vi "API Value to Temp.vi"(10 "API Temp":dbl) -> (2 "Color Temp":dbl)   [LabVIEW 2022 SP3, in "TouchControl.lvlib" / "LightsPanel.lvclass"]
uses:
  LightsPanel.lvclass
  <vilib>/Analysis/NI_AALPro.lvlib
panel:
  out "offset":dbl
  out "power":dbl
  out "amplitude":dbl
  out "Best Power Fit":dbl[](array[numeric])
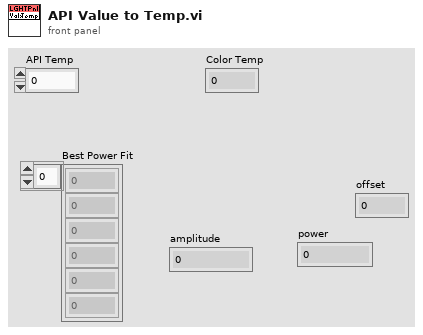
[diagram p1: front panel]
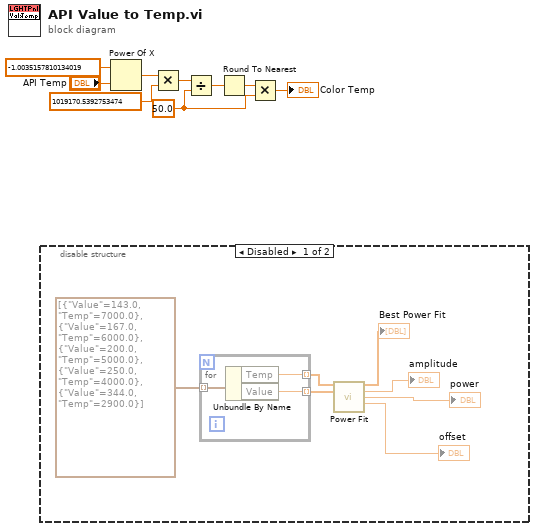
[diagram p0: block diagram]
diagram:
  w1 = 50.0 ("y")
  n1 = disable-structure shown="Disabled" {
    frame Disabled {
      n2 = for {
        tunnel: cluster{"Value":dbl, "Temp":dbl}[] [{"Value"=143.0, "Temp"=7000.0}, {"Value"=167.0, "Temp"=6000.0}, {"Value"=200.0, "Temp"=5000.0}, {"Value"=250.0, "Temp"=4000.0}, {"Value"=344.0, "Temp"=2900.0}] -> [w19] mode=indexing
        tunnel: [w18] -> w15 mode=indexing
        tunnel: [w17] -> w14 mode=indexing
        n3 = Unbundle By Name(w19) -> ("Temp"=w18:dbl, "Value"=w17:dbl)
      }
      n4 = call <vilib>:"Power Fit.vi"("Y"=w15, "X"=w14) -> ("Best Power Fit"=→"Best Power Fit":dbl[], "amplitude"=→"amplitude":dbl, "power"=→"power":dbl, "offset"=→"offset":dbl)  [unwired: 8 in, 2 out]
    }
    frame Enabled {
    }
  }
  n5 = Power Of X(1:"API Temp", 2:-1.0035157810134019 ("power")) -> (0:w5:dbl)
  n6 = Multiply(x=w5, y=1019170.5392753474) -> (x*y=w8:dbl)
  n7 = Divide(x=w8, y=w1) -> (x/y=w4:dbl)
  n8 = Round To Nearest(number=w4) -> (nearest integer value=w3:dbl)
  n9 = Multiply(x=w3, y=w1) -> (x*y=→"Color Temp":dbl)
